vi "Komponentenausgabe HovaCAL fix.vi"(8 "error in (no error)":errorcluster caption="Fehler (Eingang, kein Fehler)", 11 "Gasnummer in":T1=1 min=1 max=5) -> (0 "error out":errorcluster caption="Fehler (Ausgang)", 1 "fix":bool, 2 "Gaskomponente":T2, 3 "Gasnummer out":T1=1 min=1 max=5)   [LabVIEW 2020, in "Linearisierung v2.lvlib" / "Gasteiler.lvlib" / "HovaCAL_Interface.lvlib" / "Helper.lvlib"]
uses:
  Helper.lvlib
  Gasnumber.ctl
  Visualisierungs Elemente/Auswahlfeld.ctl
  Aktionen FGV Gasteiler Daten.ctl
  GasteilerType.ctl
  Kommunikation/Aktion FGV HovaCAL Interface Autolin.ctl
  Gasteiler.lvlib
  Linearisierung v2.lvlib
  Kommunikation/Kommunikation.lvlib
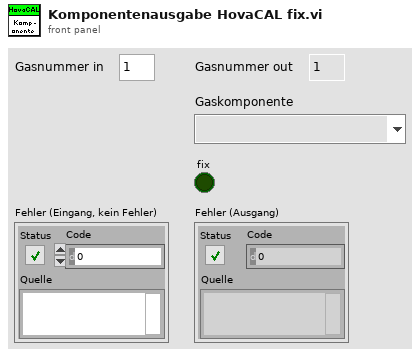
[diagram p1: front panel]
types:
  T1 = typedef "Linearisierung v2.lvlib/Gasnumber.ctl" = u8
  T2 = typedef "Auswahlfeld.ctl" = u16
  T3 = typedef "Linearisierung v2.lvlib/Gasteiler.lvlib/HovaCAL_Interface.lvlib/Kommunikation.lvlib/Aktion FGV HovaCAL Interface Autolin.ctl" = enum16{"lesen", "schreiben", "MFC Komponente fix setzen", "init"}
  T4 = typedef "Linearisierung v2.lvlib/GasteilerType.ctl" = u16
  T5 = typedef "Linearisierung v2.lvlib/Gasteiler.lvlib/Aktionen FGV Gasteiler Daten.ctl" = enum16{"lesen", "Gasteiler Daten", "Seriellen Param.", "MB-Endwert", "laden", "speichern", "Anforderung", "TCP", "Aufzeichnung Start"}
  T6 = typedef "Linearisierung v2.lvlib/Gasteiler.lvlib/Gasteiler Daten.ctl" = cluster{"Gasteiler":T7, "Gasteiler Stufen":T8, "Gasteiler Type":T4, "Konfig Gasteiler":T9, "Gasteiler Span Eingänge":u16}
  T7 = typedef "String - Eingabefeld.ctl" = string
  T8 = typedef "Linearisierung v2.lvlib/Gasteiler.lvlib/Gasteiler Stufen.ctl" = u16
  T9 = typedef "System Einstellungen V2.lvlib/Gasteiler Auswahl.ctl" = u16
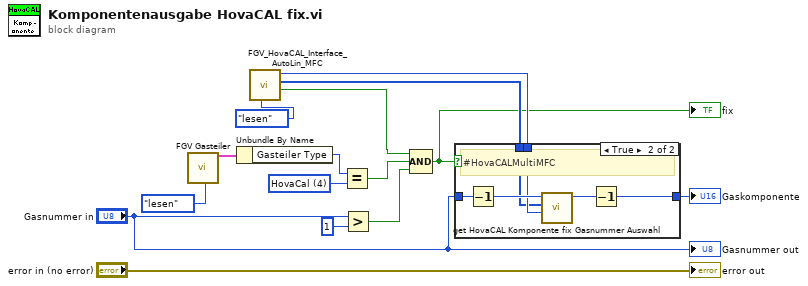
[diagram p0: block diagram]
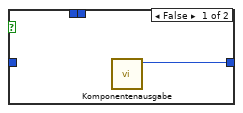
[diagram p2: hidden frame]
diagram:
  w12 = T4 4 items=["LNI", "Analog-Display", "AVL GDU", "Horiba GDC", "HovaCal", "Horiba SGD 710C"] ("y")
  n1 = call "FGV Gasteiler.vi"("Aktionen"=Aktionen_FGV_Gasteiler_Daten."lesen") -> ("Gasteiler Daten"=w11:T6)  [unwired: 11 in, 7 out]
  n2 = Unbundle By Name(w11) -> ("Gasteiler Type"=w13:T4)
  n3 = call "FGV_HovaCAL_Interface_AutoLin_MFC.vi"("Aktion"=Aktion_FGV_HovaCAL_Interface_Autolin."lesen") -> ("fix conf"=w6:bool, "MFV Komponente fix out"=w8:u16[], "AutoLin MFC out"=w9:u16)  [unwired: 7 in, 1 out]
  n4 = Equal?(x=w13, y=w12) -> (x = y?=w7:bool)
  n5 = Greater?(x="Gasnummer in", y=T1 1 ("x")) -> (0:w3:bool)
  n6 = Compound Arithmetic op=AND ("Mehrfacharithmetik")(w6, w7, w3) -> (w5:bool)
  "fix" <- w5
  n7 = case shown="True" w5 {
    tunnel: w9 -> [_ w20]
    tunnel: w8 -> [_ w19]
    tunnel: [w16 w18] -> w1
    tunnel: "Gasnummer in" -> [_ w17]
    frame False {
      n8 = call "Komponentenausgabe.vi"() -> ("Gaskomponente"=w16:T2)  [unwired: 8 in, 3 out]
    }
    frame True {
      # "#HovaCALMultiMFC"
      n9 = Decrement(x=w17) -> (x-1=w22:T1)
      n10 = call "get HovaCAL Komponente fix Gasnummer Auswahl.vi"("AutoLin MFC in"=w20, "MFV Komponente fix in"=w19, "Gasnummer EPA"=w22) -> ("MFV Komponente fix out"=w21:u16)  [unwired: 8 in]
      n11 = Decrement(x=w21) -> (x-1=w18:u16)
    }
  }
  "Gaskomponente" <- w1
  "error out" <- "error in (no error)"
  "Gasnummer out" <- "Gasnummer in"
